vi "Setup subWorker - TCP Listener.vi"(8 "error in":errorcluster, 11 "TCP Server in":refnum<class "TCP Server.lvclass">) -> (0 "error out":errorcluster, 3 "TCP Server out":refnum<class "TCP Server.lvclass">)   [LabVIEW 2017, in "_TCP Server.lvlib" / "TCP Server.lvclass"]
doc: "This VI sets up the framework parameters of a statically-linked subWorker."
uses:
  TCP Server.lvclass
  TCP Server.lvclass/TCP Server.ctl
  TCP Listener/TCP Listener.lvclass
  C:/SC/Source Code/VIPM/LabVIEW 20xx/vi.lib/addons/_Workers/Library/Classes/Worker/Worker.lvclass
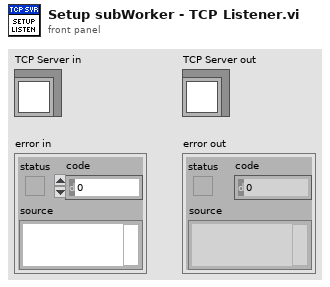
[diagram p1: front panel]
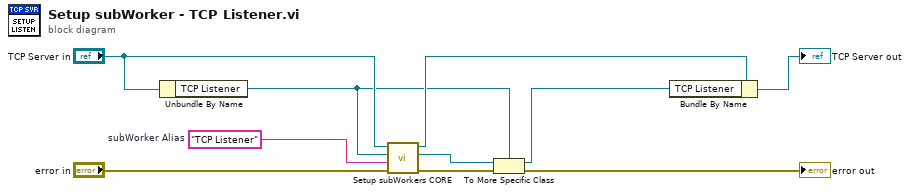
[diagram p0: block diagram]
diagram:
  w6 = "TCP Listener"  # subWorker Alias
  n1 = Unbundle By Name("TCP Server in") -> ("TCP Listener"=w3:refnum<class "TCP Listener.lvclass">)
  n2 = call-dynamic "Setup subWorkers CORE.vi"("error in"="error in", "subWorker Alias"=w6, "subWorker"=w3, "Worker"="TCP Server in") -> ("error out"=w5:errorcluster, "subWorker out"=w1:refnum<class "Worker.lvclass">, "Worker out"=w8:refnum<class "TCP Server.lvclass">)  [unwired: 5 in]
  n3 = To More Specific Class(target class=w3, reference=w1, error in=w5) -> (specific class reference=w2:refnum<class "TCP Listener.lvclass">, error out=→"error out":errorcluster)
  n4 = Bundle By Name(cluster=w8, "TCP Listener"=w2) -> (→"TCP Server out":refnum<class "TCP Server.lvclass">)
